vi "Random SubVI.vi"(11 "Alternate Stop":bool) -> ()   [LabVIEW 2016]
uses:
  Robot Global Data.vi
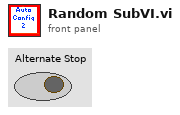
[diagram p1: front panel]
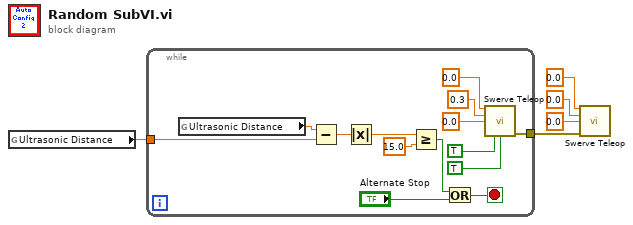
[diagram p0: block diagram]
diagram:
  n1 = global read "Robot Global Data.vi" "Ultrasonic Distance"() -> (w5:dbl)
  n2 = while {
    tunnel: [w8] -> w4
    tunnel: w5 -> [w6]
    stop <- w14 stop-if-true
    n3 = global read "Robot Global Data.vi" "Ultrasonic Distance"() -> (w7:dbl)
    n4 = Subtract(x=w7, y=w6) -> (x-y=w19:dbl)
    n5 = Absolute Value(x=w19) -> (abs(x)=w17:dbl)
    n6 = Greater Or Equal?(x=w17, y=15.0) -> (x >= y?=w16:bool)
    n7 = Or(x=w16, y="Alternate Stop") -> (x .or. y?=w14:bool)
    n8 = call "Swerve Teleop.vi"("X"=0.0, "Y"=0.3, "Z"=0.0, "Robot Centric?"=TRUE, "Autonomous?"=TRUE) -> ("Error Out"=w8:errorcluster)  [unwired: 6 in, 4 out]
  }
  n9 = call "Swerve Teleop.vi"("X"=0.0, "Y"=0.0, "Z"=0.0, "Error In"=w4) -> ()  [unwired: 7 in, 5 out]
